vi "3Act Helper - FStoPWM.vi"(11 "Suggested Rudder Setpoint in":T1 min=-1.0 max=1.0 scale=1.0..-1.0) -> (2 "freq [Hz] out":dbl, 3 "Suggested Rudder Setpoint out":T1 min=-1.0 max=1.0 scale=1.0..-1.0)   [LabVIEW 2013]
doc: "This VI is drawn directly from the MyRIO Servo example code, it's packed away in this VI for cleanup purposes. Look to the SErvo example code in the MyRIO Practice folder for debugging help. The values are directly from the example.\n\nEric Schneider, March 2014"
uses:
  Data/TypeDefs/Rudder Set Suggestions.ctl
panel:
  out "offset [%FS]":dbl
  in  "null offset":bool
  out "duty cycle [%]":dbl
  out "pulse width [ms]":dbl=1.5
  in  "freq [Hz] in":dbl=50.0
  # "Default settings from MyRIO example servo command code"
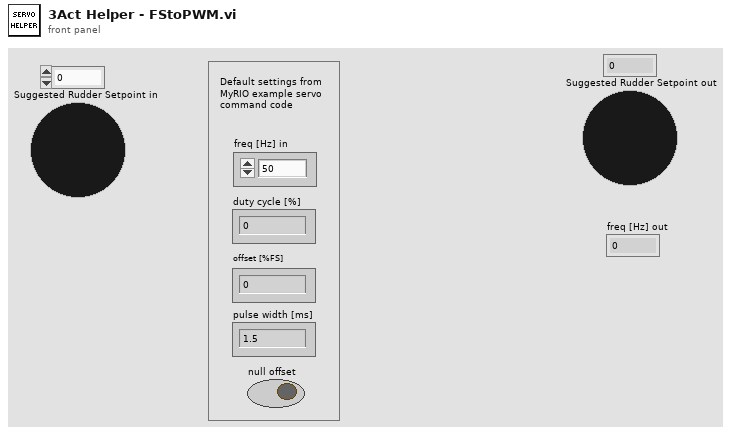
[diagram p1: front panel]
types:
  T1 = typedef "Rudder Set Suggestions.ctl" = dbl
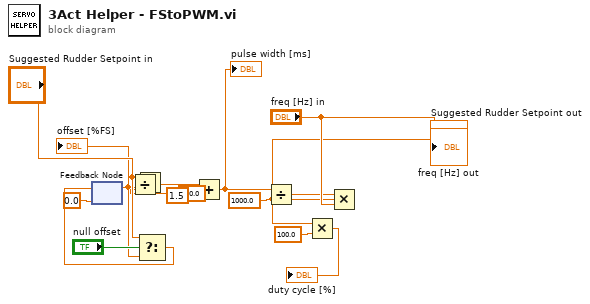
[diagram p0: block diagram]
diagram:
  n1 = feedback #1(0.0 ("position [%FS]")) -> (w6:T1)
  "offset [%FS]" <- w6
  n2 = Add(x="Suggested Rudder Setpoint in", y=w6) -> (x+y=w7:T1)
  n3 = Divide(x=w7, y=200.0) -> (x/y=w14:T1)
  n4 = Select(t="Suggested Rudder Setpoint in", s="null offset", f=w6) -> (s? t:f=w8:T1)
  n5 = feedback-in #1(w8) -> ()
  n6 = Add(x=w14, y=1.5) -> (x+y=w12:T1)
  "pulse width [ms]" <- w12
  n7 = Divide(x=w12, y=1000.0) -> (x/y=w5:T1)
  n8 = Multiply(x=w5, y="freq [Hz] in") -> (x*y=w2:T1)
  "Suggested Rudder Setpoint out" <- w2
  n9 = Multiply(x=w2, y=100.0) -> (x*y=→"duty cycle [%]":T1)
  "freq [Hz] out" <- "freq [Hz] in"
